vi "ReadObjectLayout.vi"(7 "properties to ignore":variant, 8 "error in (no error)":errorcluster, 10 "GObj Refnum":refnum<vi>, 11 "Decoration Layout in":refnum<class "Decoration Layout.lvclass">) -> (0 "error out":errorcluster, 3 "Decoration Layout out":refnum<class "Decoration Layout.lvclass">)   [LabVIEW 2010, in "NI_SE_Front Panel Layout.lvlib" / "Decoration Layout.lvclass"]
doc: "Read layout information from the GObj Refnum."
uses:
  Decoration Layout.lvclass
  Object Layout/Object Layout.lvclass
  Decoration Layout.lvclass/Decoration Layout.ctl
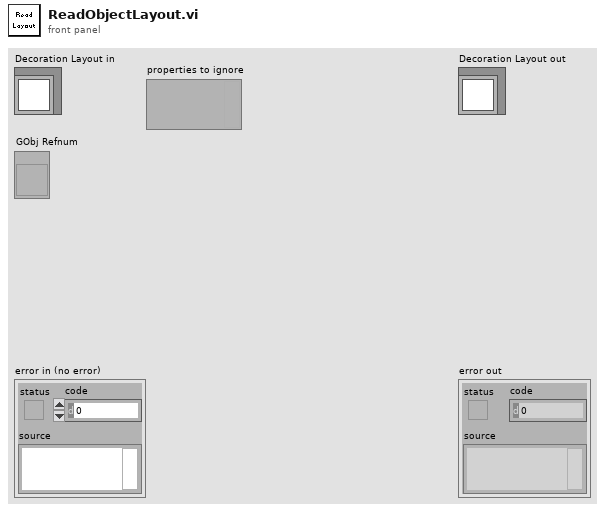
[diagram p1: front panel]
types:
  T1 = typedef "LVBoundsTypeDef.ctl" = cluster{"Width":u32, "Height":u32}
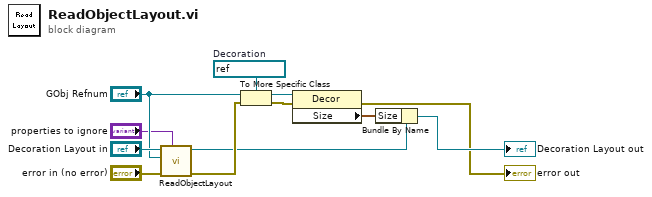
[diagram p0: block diagram]
diagram:
  w4 = refnum<vi> refnum  # Decoration
  n1 = call-parent "ReadObjectLayout.vi"("properties to ignore"="properties to ignore", "error in (no error)"="error in (no error)", "GObj Refnum"="GObj Refnum", "Object Layout in"="Decoration Layout in") -> ("error out"=w10:errorcluster, "Object Layout out"=w9:refnum<class "Decoration Layout.lvclass">)  [unwired: 6 in]
  n2 = To More Specific Class(target class=w4, reference="GObj Refnum", error in=w10) -> (specific class reference=w3:refnum<vi>, error out=w2:errorcluster)
  n3 = property class="Decor"(reference=w3, error in=w2) -> (error out=→"error out":errorcluster, "Size"=w1:T1)  [unwired: 1 out]
  n4 = Bundle By Name(cluster=w9, "Size"=w1) -> (→"Decoration Layout out":refnum<class "Decoration Layout.lvclass">)
